vi "Layout - JSON Format.vi"(8 "error in (no error)":errorcluster) -> (0 "error out":errorcluster)   [LabVIEW 2026, in "Tests.lvlib"]
doc: "Unit test (Caraya). Verifies JSONLayout.Format emits one valid JSON object per statement in slog key order (time, level, msg, then sourceTag and originVI): a full statement emits all keys, empty attributes (sourceTag/originVI) are omitted, msg is present even when empty, and message text is JSON-escaped. The timestamp is built as a fixed UTC instant with useUTC stamped TRUE so the line is deterministic (SRS-LMBR-015). Pure, no fixtures.\n\nImplements LMBR-T-005 (a-d) -> SRS-015. Assert-level IDs: Test-ID-Assert-Checklist.md."
uses:
  Tests.lvlib
  <vilib>/Utility/miscctls.llb/LVDateTimeRec.ctl
  src/TypeDefs/Statement.ctl
  src/TypeDefs/Severity.ctl
  src/Core/Layouts/JSONLayout.lvclass/JSONLayout.lvclass
  <vilib>/addons/_JKI Toolkits/Caraya/classes/Assert/Assert Equal Value_Variant.vi
  <vilib>/addons/_JKI Toolkits/Caraya/classes/Test/Test.lvclass
  <vilib>/addons/_JKI Toolkits/Caraya/classes/Assert/Assert.lvclass
  src/Lumberjack.lvlib
  src/Core/Layouts/Layout.lvclass/Layout.lvclass
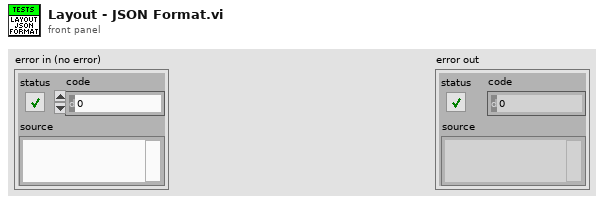
[diagram p1: front panel]
types:
  T1 = typedef "Lumberjack.lvlib/Severity.ctl" = enum16{"OFF", "FATAL", "ERROR", "WARN", "INFO", "DEBUG", "TRACE", "ALL"}
  T2 = typedef "Lumberjack.lvlib/Statement.ctl" = cluster{"timestamp":timestamp, "level":T1, "sourceTag":string, "originVI":string, "message":string}
  T3 = typedef "LVDateTimeRec.ctl" = cluster{"fractional second":dbl, "second":i32, "minute":i32, "hour":i32, "day of month":i32, "month":i32, "year":i32, "day of week":i32, "day of year":i32, "DST":i32}
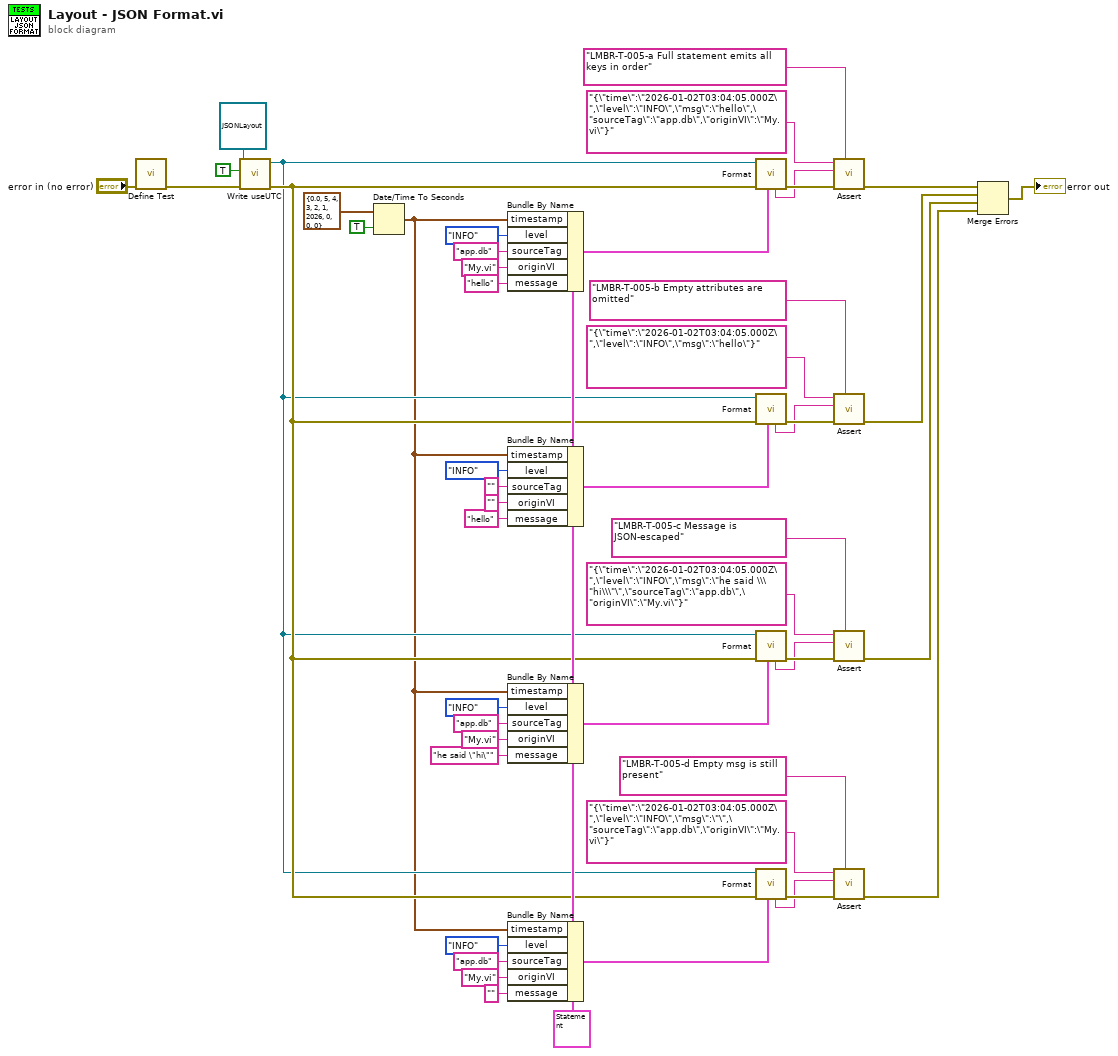
[diagram p0: block diagram]
diagram:
  w9 = T2 {"timestamp"=timestamp(0 s since 1904-01-01), "level"=enum."INFO", "sourceTag"="", "originVI"="", "message"=""} ("Statement")
  n1 = call <vilib>:"Define Test.vi"("error in (no error)"="error in (no error)") -> ("error out"=w6:errorcluster)  [unwired: 9 in, 1 out]
  n2 = call "Write useUTC.vi"("error in (no error)"=w6, "useUTC"=TRUE, "Layout in"=refnum<class "JSONLayout.lvclass"> refnum ("JSONLayout in")) -> ("error out"=w5:errorcluster, "Layout out"=w3:refnum<class "JSONLayout.lvclass">)  [unwired: 7 in]
  n3 = Date/Time To Seconds(1:TRUE ("is UTC (F)"), 2:T3 {"fractional second"=0.0, "second"=5, "minute"=4, "hour"=3, "day of month"=2, "month"=1, "year"=2026, "day of week"=0, "day of year"=0, "DST"=0} ("date time rec")) -> (0:w1:timestamp)
  n4 = Bundle By Name(cluster=w9, "timestamp"=w1, "level"=Severity."INFO", "sourceTag"="app.db", "originVI"="My.vi", "message"="hello") -> (w38:T2)
  n5 = Bundle By Name(cluster=w9, "timestamp"=w1, "level"=Severity."INFO", "sourceTag"="", "originVI"="", "message"="hello") -> (w31:T2)
  n6 = Bundle By Name(cluster=w9, "timestamp"=w1, "level"=Severity."INFO", "sourceTag"="app.db", "originVI"="My.vi", "message"="he said \"hi\"") -> (w19:T2)
  n7 = Bundle By Name(cluster=w9, "timestamp"=w1, "level"=Severity."INFO", "sourceTag"="app.db", "originVI"="My.vi", "message"="") -> (w10:T2)
  n8 = call-dynamic "Format.vi"("Statement"=w38, "error in (no error)"=w5, "JSONLayout in"=w3) -> ("error out"=w44:errorcluster, "FormattedLine"=w43:string)  [unwired: 6 in, 1 out]
  n9 = call-dynamic "Format.vi"("Statement"=w31, "error in (no error)"=w5, "JSONLayout in"=w3) -> ("error out"=w37:errorcluster, "FormattedLine"=w36:string)  [unwired: 6 in, 1 out]
  n10 = call-dynamic "Format.vi"("Statement"=w19, "error in (no error)"=w5, "JSONLayout in"=w3) -> ("error out"=w25:errorcluster, "FormattedLine"=w24:string)  [unwired: 6 in, 1 out]
  n11 = call-dynamic "Format.vi"("Statement"=w10, "error in (no error)"=w5, "JSONLayout in"=w3) -> ("error out"=w16:errorcluster, "FormattedLine"=w15:string)  [unwired: 6 in, 1 out]
  n12 = call-poly <vilib>:"Assert.vi"("Label"="LMBR-T-005-a Full statement emits all keys in order", "error in (no error)"=w44, "Actual"=w43, "Expected"="{\"time\":\"2026-01-02T03:04:05.000Z\",\"level\":\"INFO\",\"msg\":\"hello\",\"sourceTag\":\"app.db\",\"originVI\":\"My.vi\"}" ("raw")) -> ("error out"=w48:errorcluster)  [unwired: 6 in, 1 out]
  n13 = call-poly <vilib>:"Assert.vi"("Label"="LMBR-T-005-b Empty attributes are omitted", "error in (no error)"=w37, "Actual"=w36, "Expected"="{\"time\":\"2026-01-02T03:04:05.000Z\",\"level\":\"INFO\",\"msg\":\"hello\"}" ("raw")) -> ("error out"=w30:errorcluster)  [unwired: 6 in, 1 out]
  n14 = call-poly <vilib>:"Assert.vi"("Label"="LMBR-T-005-c Message is JSON-escaped", "error in (no error)"=w25, "Actual"=w24, "Expected"="{\"time\":\"2026-01-02T03:04:05.000Z\",\"level\":\"INFO\",\"msg\":\"he said \\\"hi\\\"\",\"sourceTag\":\"app.db\",\"originVI\":\"My.vi\"}" ("raw")) -> ("error out"=w8:errorcluster)  [unwired: 6 in, 1 out]
  n15 = call-poly <vilib>:"Assert.vi"("Label"="LMBR-T-005-d Empty msg is still present", "error in (no error)"=w16, "Actual"=w15, "Expected"="{\"time\":\"2026-01-02T03:04:05.000Z\",\"level\":\"INFO\",\"msg\":\"\",\"sourceTag\":\"app.db\",\"originVI\":\"My.vi\"}" ("raw")) -> ("error out"=w7:errorcluster)  [unwired: 6 in, 1 out]
  n16 = Merge Errors(w48, w30, w8, w7) -> (→"error out":errorcluster)
